vi "Binary File Create using Boolean.vi"() -> ()   [LabVIEW 2015]
panel:
  out "Array":bool[](array[boolean])
  out "unsigned 8bit integer":u8
  in  "file path (use dialog)":path
  # "Binary File Create using Boolean"
  # "Pardeep Kumar"
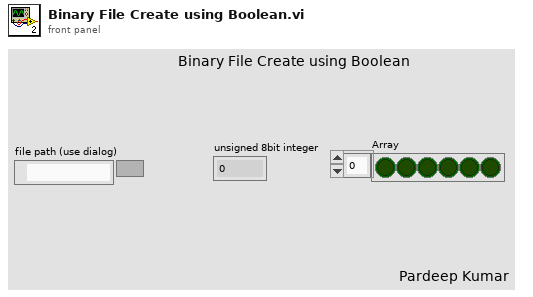
[diagram p1: front panel]
types:
  T1 = enum16{"open", "replace", "create", "open or create", "replace or create", "replace or create with confirmation"}
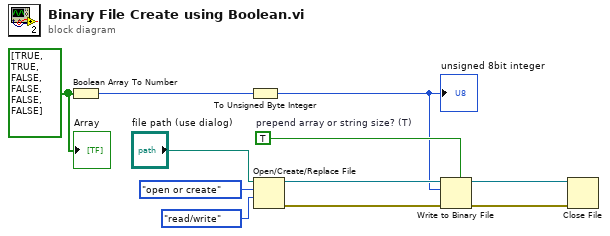
[diagram p0: block diagram]
diagram:
  w3 = bool[] [TRUE, TRUE, FALSE, FALSE, FALSE, FALSE]
  w4 = TRUE  # prepend array or string size? (T)
  n1 = Boolean Array To Number(Boolean array=w3) -> (number=w2:u32)
  n2 = To Unsigned Byte Integer(number=w2) -> (unsigned 8bit integer=w1:u8)
  "unsigned 8bit integer" <- w1
  n3 = Open/Create/Replace File(file path (use dialog)="file path (use dialog)", operation (0:open)=T1."open or create", access (0:read/write)=enum16{"read/write", "read-only", "write-only"}."read/write") -> (refnum out=w11:refnum<file>, error out=w9:errorcluster)  [unwired: 3 in, 1 out]
  n4 = Write to Binary File(file (use dialog)=w11, data=w1, error in=w9, 5:w4) -> (refnum out=w10:refnum<file>, error out=w8:errorcluster)  [unwired: 2 in, 1 out]
  n5 = Close File(refnum=w10, error in=w8) -> ()  [unwired: 2 out]
  "Array" <- w3
